vi "Select_Data.vi"(2 "Desired Signal":enum16{"Raw", "Env"}(ring), 3 "Cluster":cluster{"all rows":dbl[][], i32, dbl}) -> (0 "Signal Sequence":dbl[](array[numeric]), 1 "Waveform":waveform(dbl))   [LabVIEW 2019]
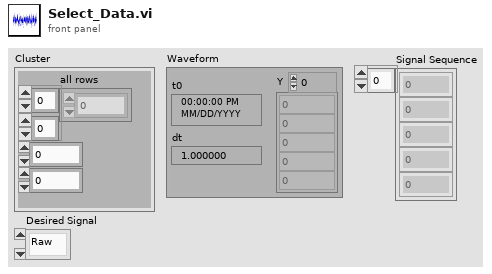
[diagram p1: front panel]
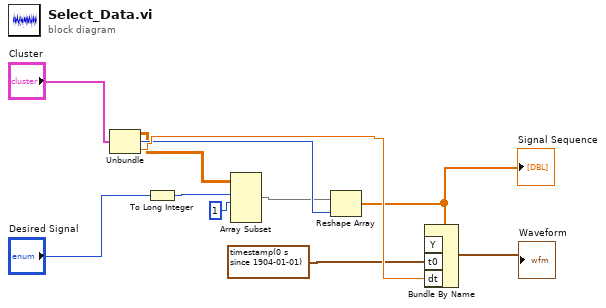
[diagram p0: block diagram]
diagram:
  n1 = Unbundle("Cluster") -> ("all rows"=w9:dbl[][], w10:i32, w11:dbl)
  n2 = To Long Integer(number="Desired Signal") -> (32bit integer=w3:i32)
  n3 = Array Subset(array=w9, index (row)=w3, length (row)=1 ("length")) -> (w2:dbl[][])  [unwired: 2 in]
  n4 = Reshape Array(w2, w10) -> (w1:dbl[])
  "Signal Sequence" <- w1
  n5 = Bundle By Name("Y"=w1, "t0"=timestamp(0 s since 1904-01-01), "dt"=w11) -> (→"Waveform":waveform(dbl))  [unwired: 1 in]
